vi "set_instruments (SubVI).vi"(0 "Process list":T4, 1 "Flash lamp settings:":T3={"Output channel (for flashing)"="Dev4/ao0", "Loop iteration"=0, "Path"=path "", "Flash lamp\n settings:"={"Flash lamp?"=FALSE, "Number of cyles\nbetween flashes"=3, "# Pulses"=35, "Stop flashing \nbelow thresh?"=FALSE, "Stop threshold"=0.001, "Pulse voltage?"=FALSE, "Pulse length (ms)"=0.001, "Pulse amp (V)"=0.001}}, 4 "electrodes reference":refnum<vi>, 5 "instrument config":T2, 6 "Num samples":i32, 7 "small amp":dbl=1.0 format="%0.2p", 9 "Volt vs pos array":cluster{dbl, dbl}[](array[cluster]), 10 "wfm?":bool, 11 "small amp freq":dbl=10.0 format="%0.2p", 12 "User Def. Wfm Name":string="RANDFREQ", 13 "Add small amp?":bool) -> (14 "Curr threshold":dbl, 18 "DC volts arr":dbl[](array[numeric]), 19 "instrum out":T1)   [LabVIEW 2014]
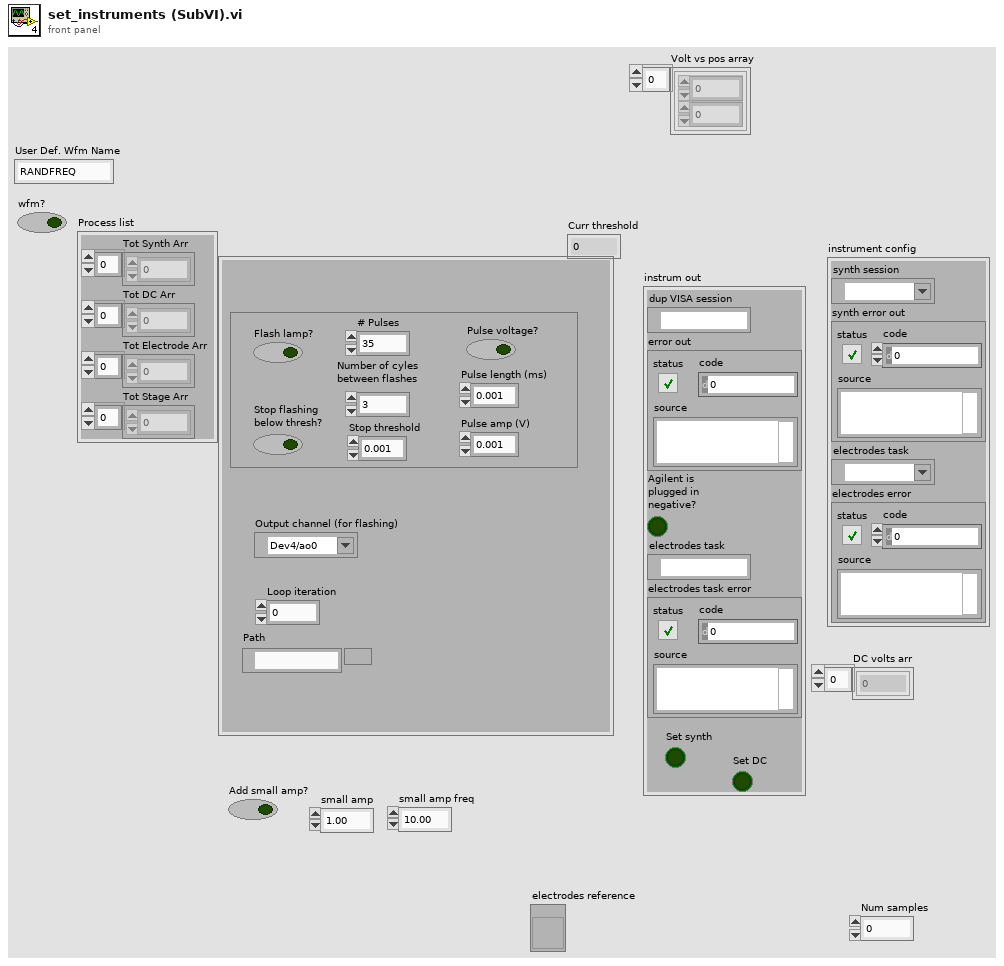
[diagram p1: front panel]
types:
  T1 = cluster{"dup VISA session":refnum<visa-resource-name>, "error out":errorcluster, "Agilent is \nplugged in \nnegative?":bool, "electrodes task":refnum<k21>, "electrodes task error":errorcluster, "Set synth":bool, "Set DC":bool}
  T2 = cluster{"synth session":refnum<visa-resource-name>, "synth error out":errorcluster, "electrodes task":refnum<k21>, "electrodes error":errorcluster}
  T3 = cluster{"Output channel (for flashing)":tag, "Loop iteration":i32, "Path":path, "Flash lamp\n settings:":cluster{"Flash lamp?":bool, "Number of cyles\nbetween flashes":i32, "# Pulses":i32, "Stop flashing \nbelow thresh?":bool, "Stop threshold":dbl, "Pulse voltage?":bool, "Pulse length (ms)":dbl, "Pulse amp (V)":dbl}}
  T4 = cluster{"Tot Synth Arr":dbl[], "Tot DC Arr":dbl[], "Tot Electrode Arr":dbl[], "Tot Stage Arr":dbl[]}
  T5 = cluster{"Flash lamp?":bool, "Number of cyles\nbetween flashes":i32, "# Pulses":i32, "Stop flashing \nbelow thresh?":bool, "Stop threshold":dbl, "Pulse voltage?":bool, "Pulse length (ms)":dbl, "Pulse amp (V)":dbl}
  T6 = cluster{"dup VISA session":refnum<visa-resource-name>, "error out":errorcluster, "Agilent is \nplugged in \nnegative?":bool, "electrodes task 2":refnum<k21>, "electrodes task error 2":errorcluster, "Set synth?":bool, "Set DC?":bool}
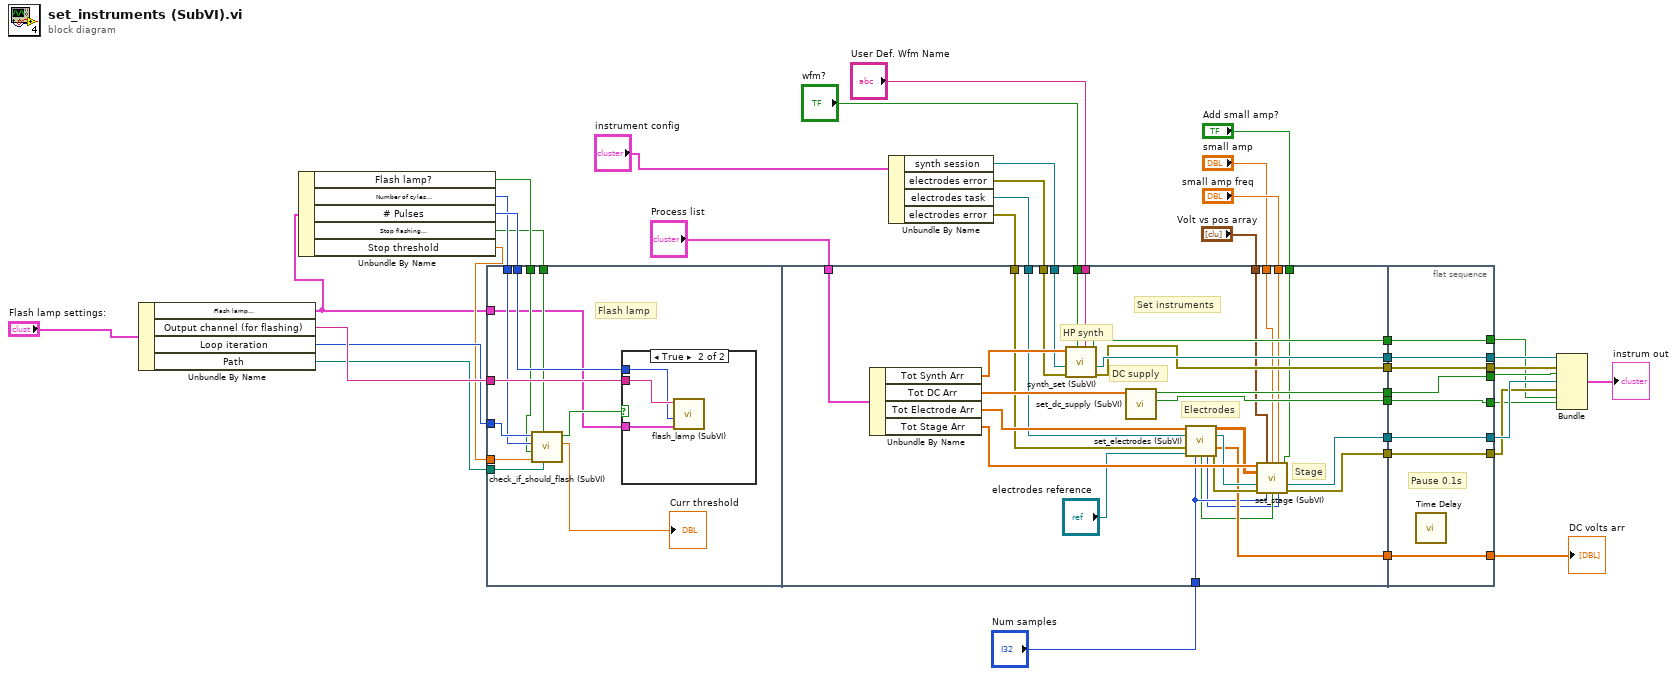
[diagram p0: block diagram]
diagram:
  n1 = Unbundle By Name("Flash lamp settings:") -> ("Flash lamp\n settings:"=w1:T5, "Output channel (for flashing)"=w38:tag, "Loop iteration"=w36:i32, "Path"=w33:path)
  n2 = Unbundle By Name(w1) -> ("Flash lamp?"=w34:bool, "Number of cyles\nbetween flashes"=w35:i32, "# Pulses"=w37:i32, "Stop flashing \nbelow thresh?"=w31:bool, "Stop threshold"=w32:dbl)
  n3 = flat-sequence {
    tunnel: w38 -> [w51]
    tunnel: w37 -> [w50]
    tunnel: w36 -> [w49]
    tunnel: w35 -> [w48]
    tunnel: w34 -> [w47]
    tunnel: w33 -> [w46]
    tunnel: w32 -> [w45]
    tunnel: w31 -> [w44]
    tunnel: w1 -> [w41]
    tunnel: "Process list" -> [w84]
    tunnel: w30 -> [w82]
    tunnel: w29 -> [w81]
    tunnel: w26 -> [w78]
    tunnel: w27 -> [w77]
    tunnel: [w67] -> w19
    tunnel: [w76] -> w18
    tunnel: [w75] -> w17
    tunnel: [w74] -> w16
    tunnel: [w66] -> w15
    tunnel: [w72] -> w14
    tunnel: [w71] -> w12
    tunnel: [w64] -> w10
    tunnel: "Num samples" -> [w63]
    tunnel: "wfm?" -> [w62]
    tunnel: "User Def. Wfm Name" -> [w61]
    tunnel: "small amp freq" -> [w58]
    tunnel: "small amp" -> [w56]
    tunnel: "Add small amp?" -> [w57]
    tunnel: "Volt vs pos array" -> [w55]
    tunnel: [w88] -> w21
    tunnel: [w89] -> w23
    tunnel: [w90] -> w24
    tunnel: [w91] -> w25
    tunnel: [w92] -> w22
    tunnel: w19 -> [w92]
    tunnel: w18 -> [w91]
    tunnel: w17 -> [w90]
    tunnel: w16 -> [w89]
    tunnel: w15 -> [w88]
    tunnel: w14 -> [w87]
    tunnel: [w87] -> w13
    tunnel: [w86] -> w11
    tunnel: w12 -> [w86]
    tunnel: [w85] -> w9
    tunnel: w10 -> [w85]
    frame #0 {
      # "Flash lamp"
      n4 = call "check_if_should_flash (SubVI).vi"("Path"=w46, "Stop below threshold"=w44, "Stop threshold"=w45, "Flash lamp?"=w47, "Number of cyles\nbetween flashes"=w48, "Loop iteration"=w49) -> ("Curr threshold"=→"Curr threshold":dbl, "Should flash"=w43:bool)  [unwired: 4 in]
      n5 = case shown="True" w43 {
        tunnel: w51 -> [_ w54]
        tunnel: w50 -> [_ w53]
        tunnel: w41 -> [_ w52]
        frame False {
        }
        frame True {
          n6 = call "flash_lamp (SubVI).vi"("Flash lamp\n settings:"=w52, "# Pulses in"=w53, "Output channel (for flashing)"=w54) -> ()  [unwired: 9 in]
        }
      }
    }
    frame #1 {
      # "Stage"
      # "Electrodes"
      # "DC supply"
      # "HP synth"
      # "Set instruments"
      n7 = Unbundle By Name(w84) -> ("Tot Synth Arr"=w83:dbl[], "Tot DC Arr"=w80:dbl[], "Tot Electrode Arr"=w79:dbl[], "Tot Stage Arr"=w73:dbl[])
      n8 = call "synth_set (SubVI).vi"("User Def. Wfm Name"=w61, "wfm?"=w62, "error in (no error)"=w81, "VISA session"=w82, "Tot Synth Arr"=w83) -> ("error out"=w75:errorcluster, "dup VISA session"=w76:refnum<visa-resource-name>, "Set synth?"=w71:bool)  [unwired: 4 in]
      n9 = call "set_dc_supply (SubVI).vi"("Tot DC Arr"=w80) -> ("Set DC?"=w72:bool, "Agilent is \nplugged in \nnegative?"=w74:bool)  [unwired: 9 in]
      n10 = call "set_electrodes (SubVI).vi"("Tot Electrode Arr"=w79, "electrodes task 2"=w78, "electrodes error"=w77, "electrodes reference"="electrodes reference", "Num samples"=w63) -> ("electrode arr"=w70:dbl[][], "electrodes task"=w69:refnum<k21>, "DC volts arr"=w64:dbl[], "Use arbitrary\nforce func?"=w60:bool, "Electrode to sweep:"=w59:i32, "electrodes task error"=w68:errorcluster)  [unwired: 5 in]
      n11 = call "set_stage (SubVI).vi"("Tot Stage Arr"=w73, "Volt vs pos array"=w55, "small amp"=w56, "small amp freq"=w58, "Add small amp?"=w57, "electrode arr"=w70, "electrodes task"=w69, "electrodes task error"=w68, "Num samples"=w63, "Use arb force?"=w60, "Electrode to sweep"=w59) -> ("electrodes task 2"=w67:refnum<k21>, "electrodes task error 2"=w66:errorcluster)  [unwired: 3 in]
    }
    frame #2 {
      # "Pause 0.1s"
      n12 = call "Time Delay"() -> ()  [unwired: 11 in, 1 out]
    }
  }
  n13 = Unbundle By Name("instrument config") -> ("synth session"=w30:refnum<visa-resource-name>, "electrodes error"=w29:errorcluster, "electrodes task"=w26:refnum<k21>, "electrodes error"=w27:errorcluster)
  n14 = Bundle("dup VISA session"=w25, "error out"=w24, "Agilent is \nplugged in \nnegative?"=w23, "electrodes task 2"=w22, "electrodes task error 2"=w21, "Set synth?"=w11, "Set DC?"=w13) -> (→"instrum out":T6)  [unwired: 1 in]
  "DC volts arr" <- w9
